vi "sub_vi_arduino_first_communication.vi"(5 "Reads number":i32, 7 "Writes number":i32, 8 "error in (no error)":errorcluster, 9 "write buffer":string, 11 "VISA resource name in":refnum<visa-resource-name>) -> (0 "error out":errorcluster, 1 "Reads array":dbl[](array[numeric]), 2 "Received data":string[](array[string]), 3 "VISA resource name out":refnum<visa-resource-name>)   [LabVIEW 2019]
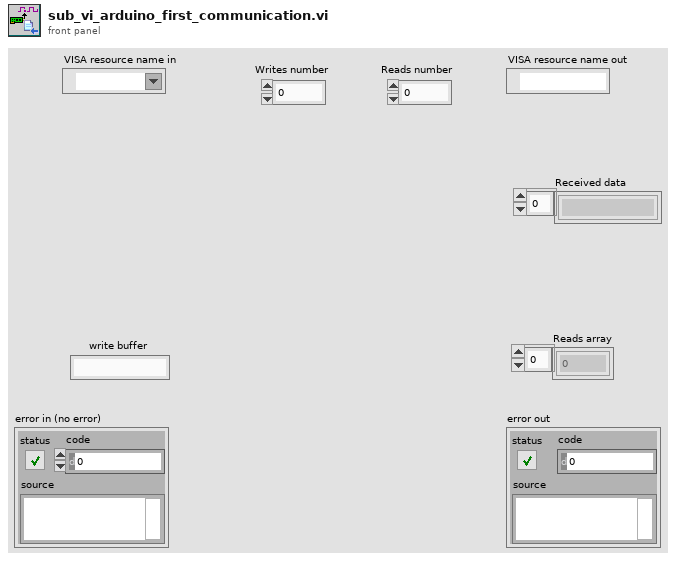
[diagram p1: front panel]
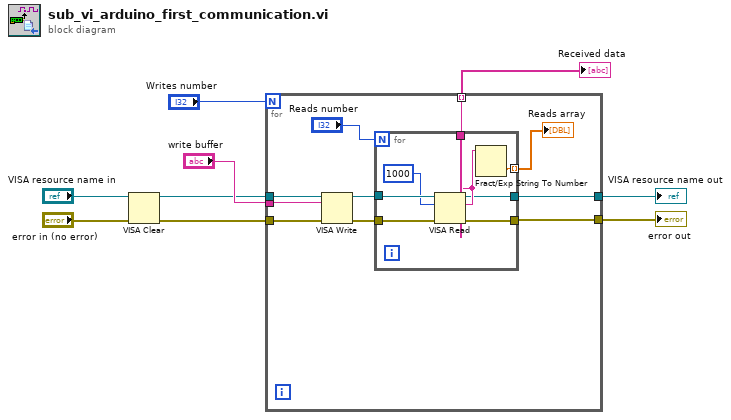
[diagram p0: block diagram]
diagram:
  n1 = VISA Clear(VISA resource name="VISA resource name in", error in (no error)="error in (no error)") -> (VISA resource name out=w5:refnum<visa-resource-name>, error out=w3:errorcluster)
  n2 = for {
    N: "Writes number" -> [_]
    tunnel: [w12] -> w8
    tunnel: [w14] -> w9
    tunnel: w3 -> [w19]
    tunnel: "write buffer" -> [w18]
    tunnel: w5 -> [w17]
    tunnel: [w13] -> w2 mode=indexing
    n3 = VISA Write(VISA resource name=w17, write buffer=w18, error in (no error)=w19) -> (VISA resource name out=w15:refnum<visa-resource-name>, error out=w16:errorcluster)  [unwired: 1 out]
    n4 = for {
      N: "Reads number" -> [_]
      tunnel: w16 -> [w26]
      tunnel: w15 -> [w25]
      tunnel: [w24] -> w14
      tunnel: [w23] -> w13
      tunnel: [w22] -> w12
      tunnel: [w20] -> w11 mode=indexing
      n5 = VISA Read(VISA resource name=w25, byte count=u32 1000, error in (no error)=w26) -> (VISA resource name out=w22:refnum<visa-resource-name>, read buffer=w23:string, error out=w24:errorcluster)  [unwired: 1 out]
      n6 = Fract/Exp String To Number(string=w23) -> (number=w20:dbl)  [unwired: 3 in, 1 out]
    }
    "Reads array" <- w11
  }
  "error out" <- w9
  "VISA resource name out" <- w8
  "Received data" <- w2
